vi "VeriStand Framework.Read.vi"(8 "error in (no error)":errorcluster, 10 "Data Ref":T1, 11 "VeriStand DSF in":refnum<class "VeriStand DSF.Framework.lvclass">=refnum) -> (0 "error out":errorcluster, 3 "VeriStand DSF out":refnum<class "VeriStand DSF.Framework.lvclass">)   [LabVIEW 2017, in "Data Sharing Custom Device Engine.lvlib" / "VeriStand DSF.Framework.lvclass"]
uses:
  VeriStand DSF.Framework.lvclass
  <vilib>/NI Veristand/Custom Device API/Data Table Ref.ctl
  Builds/Data Sharing Framework/Current/Data Sharing Framework Core/DSF Core.lvlibp/Engine/Classes/Framework/Framework.lvclass
  C:/Builds/Data Sharing Framework/Current/Data Sharing Framework Core/DSF Core.lvlibp/Engine/Classes/Framework/Framework.lvclass
  <vilib>/NI Veristand/Custom Device API/Custom Device API.lvlib
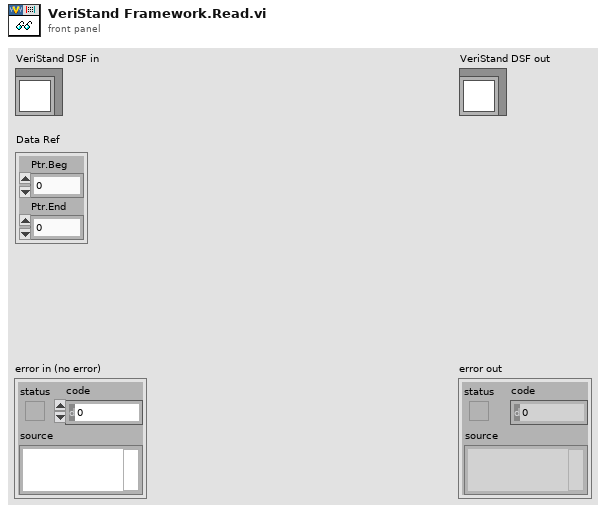
[diagram p1: front panel]
types:
  T1 = typedef "Custom Device API.lvlib/Data Table Ref.ctl" = cluster{"Ptr.Beg":u64, "Ptr.End":u64}
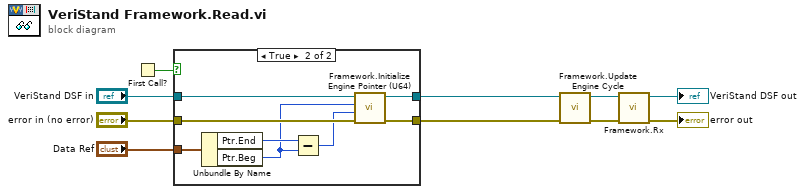
[diagram p0: block diagram]
diagram:
  n1 = First Call?() -> (First Call?: T/F=w6:bool)
  n2 = case shown="True" w6 {
    tunnel: "VeriStand DSF in" -> [w12 w16]
    tunnel: "error in (no error)" -> [w11 w15]
    tunnel: [w12 w18] -> w3
    tunnel: [w11 w17] -> w2
    tunnel: "Data Ref" -> [_ w20]
    frame False {
    }
    frame True {
      n3 = Unbundle By Name(w20) -> ("Ptr.End"=w19:u64, "Ptr.Beg"=w13:u64)
      n4 = Subtract(x=w19, y=w13) -> (x-y=w14:u64)
      n5 = call "Framework.Initialize Engine Pointer (U64).vi"("error in (no error)"=w15, "size"=w14, "address"=w13, "Framework in"=w16) -> ("error out"=w17:errorcluster, "Framework out"=w18:refnum<class "VeriStand DSF.Framework.lvclass">)  [unwired: 6 in]
    }
  }
  n6 = call-dynamic "Framework.Update Engine Cycle.vi"("error in (no error)"=w2, "Framework in"=w3) -> ("error out"=w8:errorcluster, "Framework out"=w10:refnum<class "VeriStand DSF.Framework.lvclass">)  [unwired: 8 in]
  n7 = call "Framework.Rx.vi"("error in (no error)"=w8, "Framework in"=w10) -> ("error out"=→"error out":errorcluster, "Framework out"=→"VeriStand DSF out":refnum<class "VeriStand DSF.Framework.lvclass">)  [unwired: 8 in]
